vi "AddTimeToTDMS.vi"(8 "error in":errorcluster, 11 "data":waveform(dbl)[](array[waveform])) -> (0 "error out":errorcluster, 3 "Data out":waveform(dbl)[](array[waveform]))   [LabVIEW 2019, in "DAQ.lvclass"]
uses:
  DAQ.lvclass
panel:
  out "output waveform":waveform(dbl)
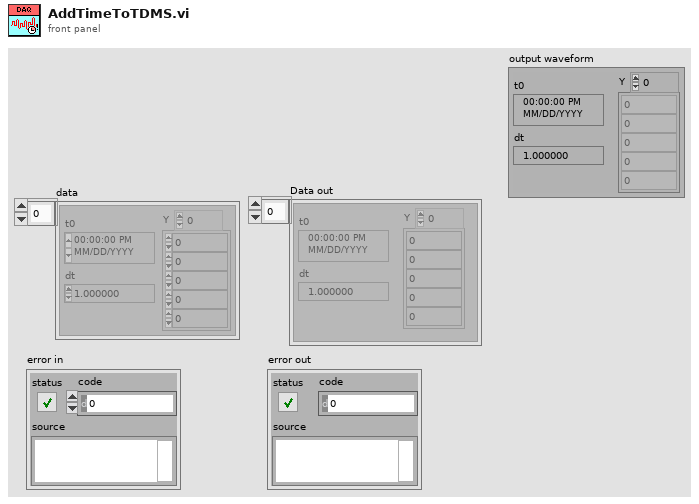
[diagram p1: front panel]
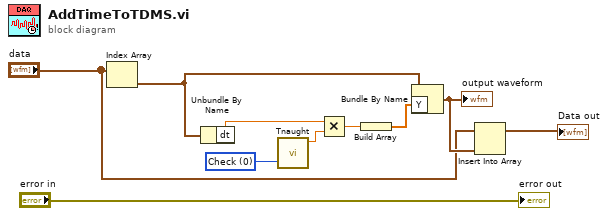
[diagram p0: block diagram]
diagram:
  w3 = u16 0 items=["Check", "Init"] ("Ring")
  n1 = Index Array(array="data") -> (element=w7:waveform(dbl))  [unwired: 1 in]
  n2 = Unbundle By Name(w7) -> ("dt"=w6:dbl)
  n3 = call "Tnaught.vi"("Ring"=w3) -> ("Numeric"=w4:dbl)  [unwired: 10 in]
  n4 = Multiply(x=w6, y=w4) -> (x*y=w2:dbl)
  n5 = Build Array(w2) -> (w1:dbl[])
  n6 = Bundle By Name(cluster=w7, "Y"=w1) -> (w10:waveform(dbl))
  "output waveform" <- w10
  n7 = Insert Into Array(array="data", new element=w10) -> (→"Data out":waveform(dbl)[])  [unwired: 1 in]
  "error out" <- "error in"
